vi "WLC fitting_twoside_slope_YCC.vi"(4 "QPD-y":dbl[](array[numeric]), 5 "QPD-x":dbl[](array[numeric]), 6 "Xstage":dbl[](array[numeric]), 7 "T=Read data mode?\nF=Real time fit":bool=TRUE) -> ()   [LabVIEW 2014]
doc: "This VI utilizes the LabVIEW implemented non-linear curve fitting algorithm to fit worm-like chain model. \nThere are 2 modes can be selected: one is real-time fitting mode, the other is data reading mode. \n\nIn the real-time fitting mode, the force-extension assay VI will automatically pass the data and the settings into this VI, and then fitting. \n\nIn the data reading mode, you should first select the data path to read, and manually input all the setting, such as height and fitting range, and then push the \"run\" button. \n\nThe VI will calculate the DNA extension, and extract the pre-set fitting range to do WLC fitting. The data output includes contour length, persistence length, fitted center, recorded data and fitted data."
uses:
  <vilib>/gmath/NI_Gmath.lvlib
  <vilib>/Utility/file.llb/Read From Spreadsheet File (DBL).vi
  <vilib>/Utility/file.llb/Write To Spreadsheet File (DBL).vi
  <vilib>/gmath/NumericalOptimization/Nonlinear Curve Fit LM formula string.vi
panel:
  out "QPD height":dbl
  in  "initial parameters for fit K":dbl[](array[numeric])=[40.0, 1150.0]
  in  "initial parameters 2":dbl[](array[numeric])=[40.0, 1150.0]
  in  "Enum":T1(ring)
  out "residue":dbl
  in  "Tab Control 2":enum32{"Page 1"}(tab)
  in  "T=positive (RHS)\nF=negative (LHS)":bool
  in  "fit only one side?":bool
  in  "OK to fit?":bool
  in  "trap height(nm)":dbl=300.0
  in  "X=T,Y=F":bool=TRUE
  in  "Tab Control":T2(tab)
  out "XY Graph 2":T3(graph)
  out "XY Graph 4":T3(graph)
  out "XY Graph":cluster{"Y":dbl[], "Y":dbl[]}[](graph)
  out "XY Graph 3":cluster{"xDNA-cut":dbl[], "Force-cut":dbl[]}[](graph)
  in  "laser power (mW)":dbl=10.0
  in  "xDNA cut outside (nm)":dbl=2000.0
  in  "stop to save?":bool
  out "yr":dbl
  out "conversion factor (V/um)":dbl=2.6
  in  "center position shift (nm)":dbl=0.0001 format="%_6g"
  in  "center QPD shift mV)":dbl=0.0001 format="%_6g"
  in  "initial parameters for marko":dbl[](array[numeric])=[40.0, 1800.0, 0.001, 0.001]
  out "yi":dbl
  out "Position Array Out":dbl[](array[numeric])
  out "Force constant (pN/nm)":dbl=0.0154
  in  "Length offset":dbl=400.0
  in  "Force offset":dbl=4.0
  in  "F-x data":path
  out "ci":dbl
  out "cr":dbl
  in  "Save fit?":bool
  out "QPD signal Out":dbl[](array[numeric])
  out "position-QPD":T4(graph)
  in  "bead radius(nm)":dbl=515.0
  out "best fit parameters":dbl[](array[numeric])
  # "Lp"
  # "L0"
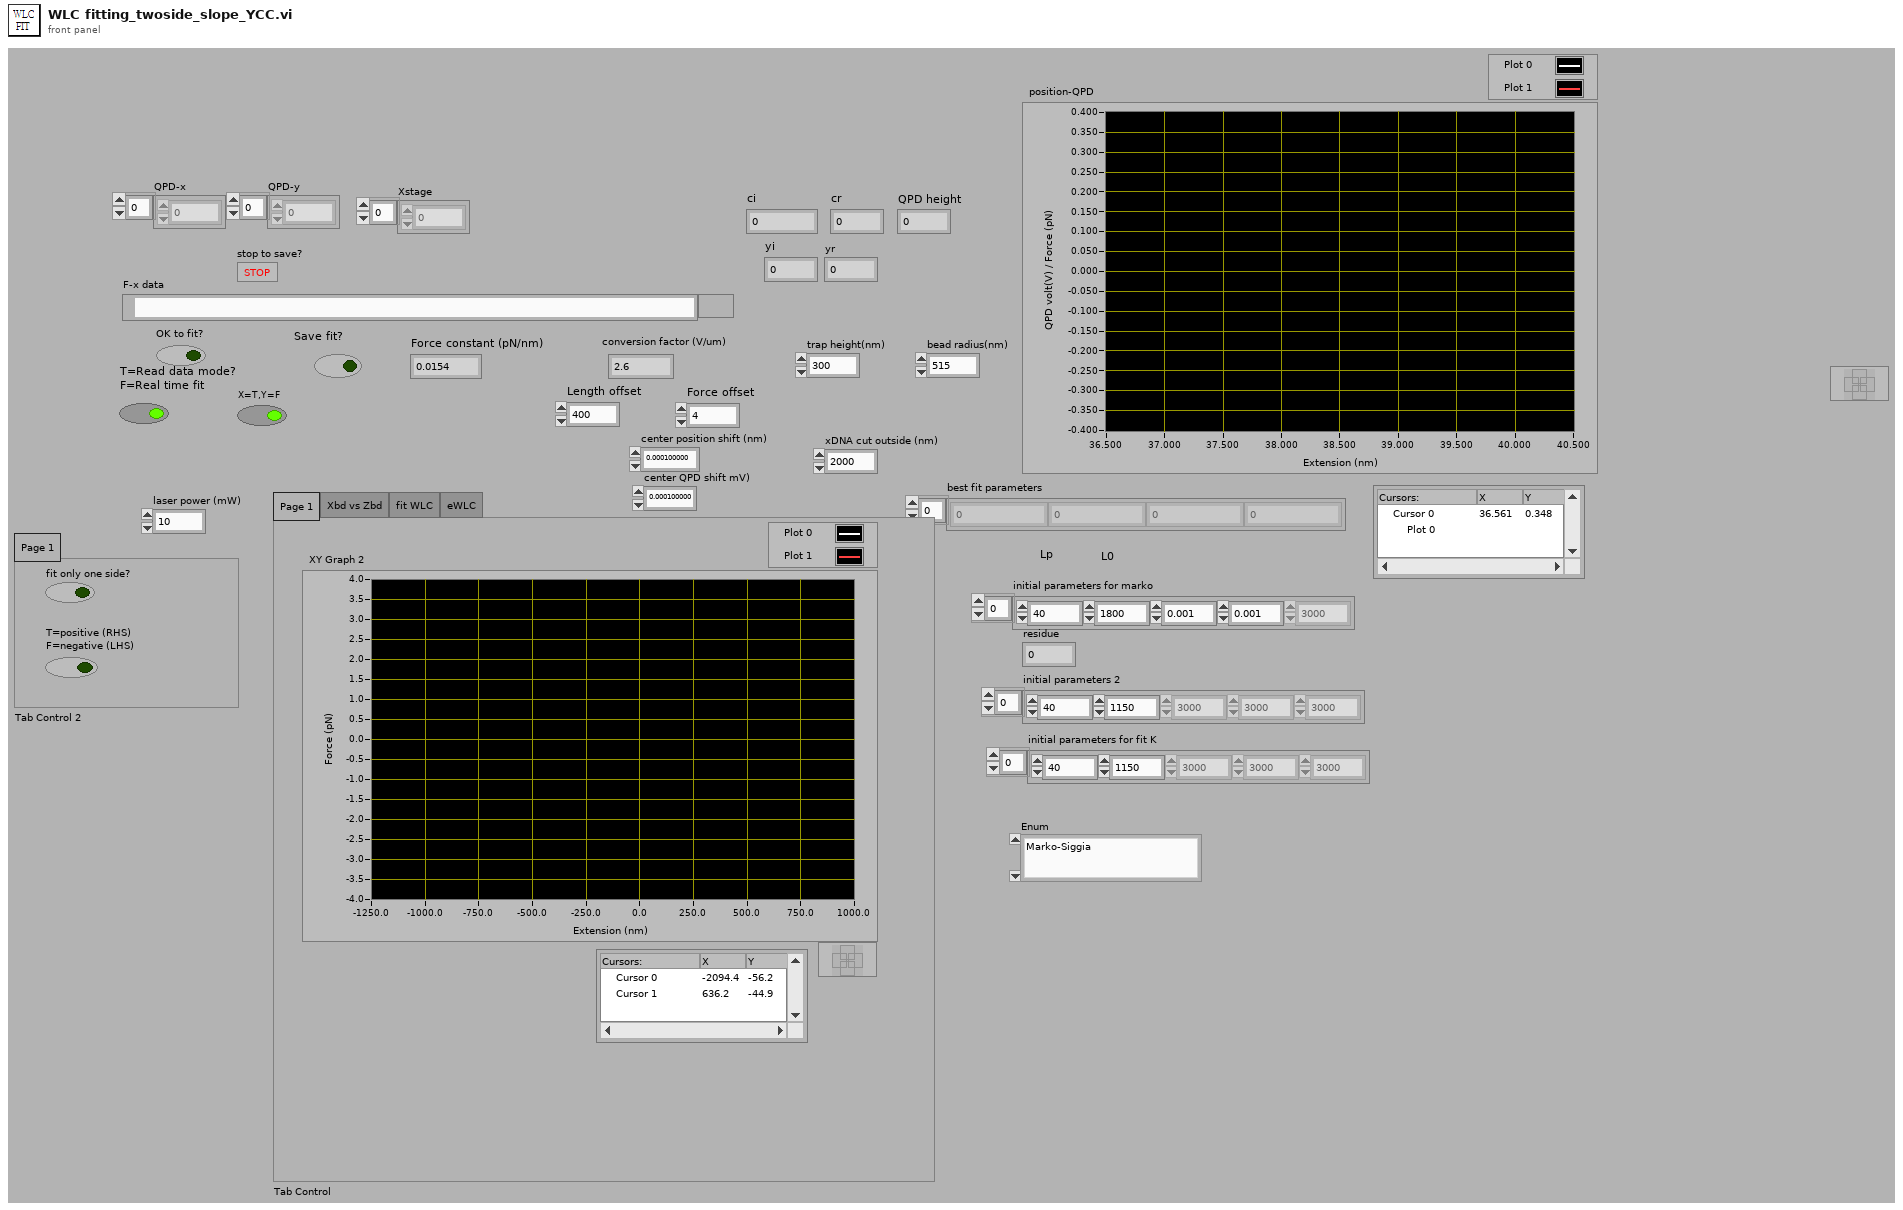
[diagram p1: front panel]
types:
  T1 = enum16{"Marko-Siggia", "modified Marko", "eWLC", "eWLC-modified M-S", "K fit eWLC-modified M-S"}
  T2 = enum32{"Page 1", "Xbd vs Zbd", "fit WLC", "eWLC"}
  T3 = cluster{"cut-full xDNA":dbl[], "cut-full Force":dbl[]}
  T4 = cluster{"QPD signal Out":dbl[], "Position Array Out":dbl[]}
  T5 = cluster{"Position Array Out":dbl[], "QPD signal Out":dbl[]}
  T6 = cluster{"model":string, "Parameters":string[], "x":string}
  T7 = cluster{"xDNA-cut":dbl[], "best nonlinear fit":dbl[]}
  T8 = cluster{"best nonlinear fit":dbl[], "Force-cut":dbl[]}
  T9 = cluster{"xDNA-cut":dbl[], "best nonlinear fit":dbl[]}[]
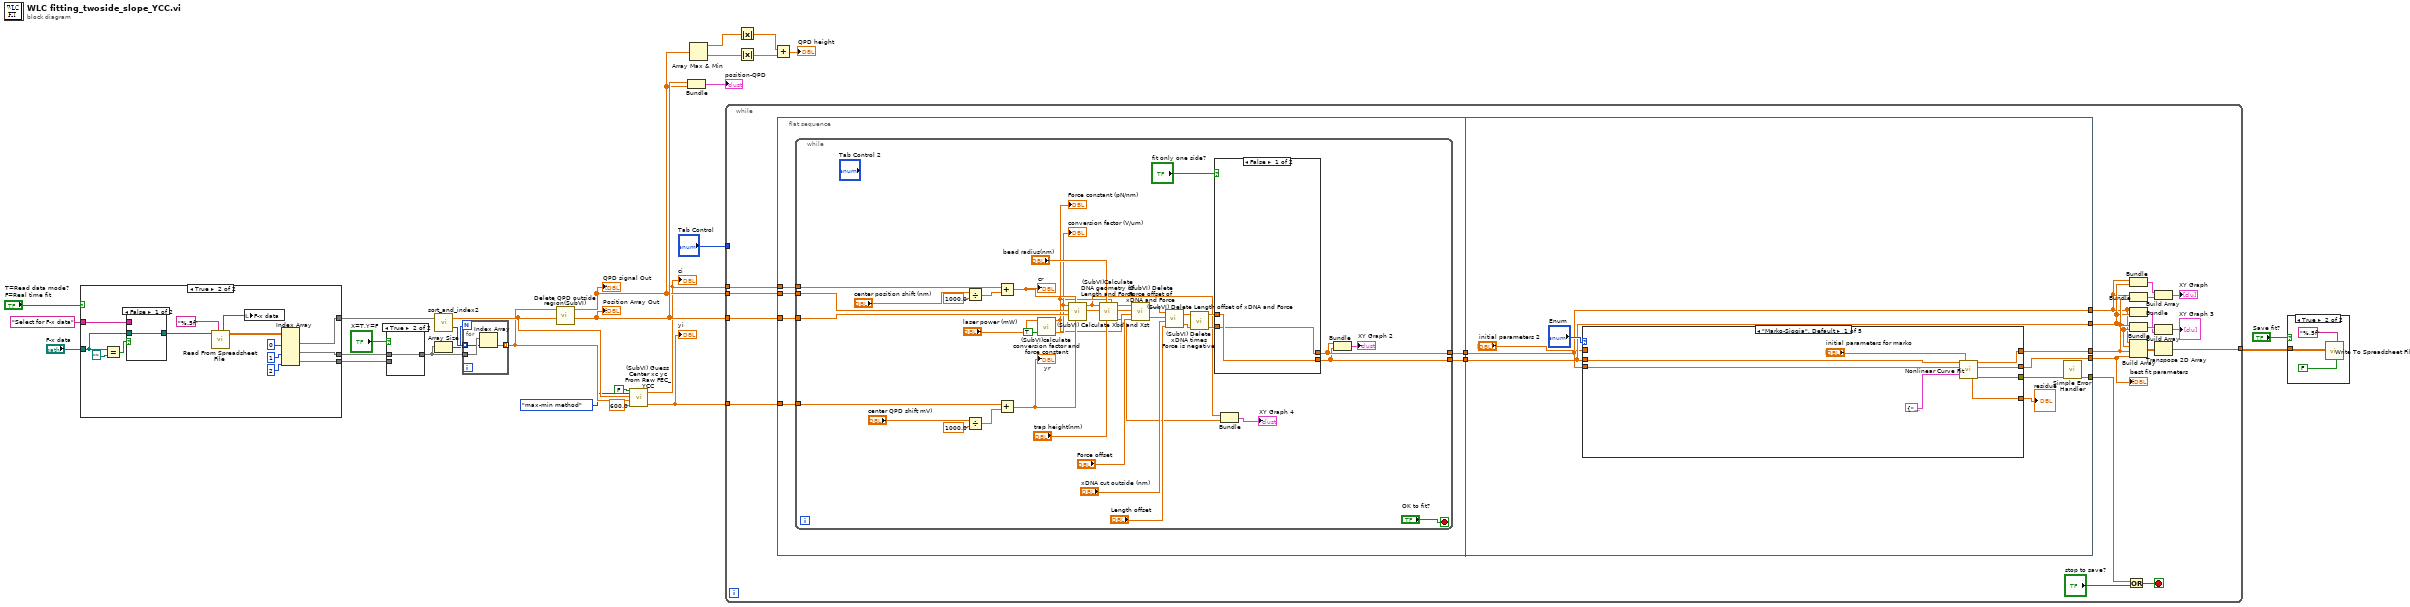
[diagram p0: block diagram]
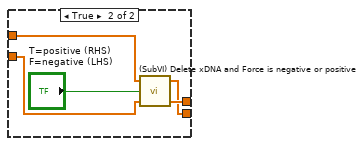
[diagram p2: hidden frame]
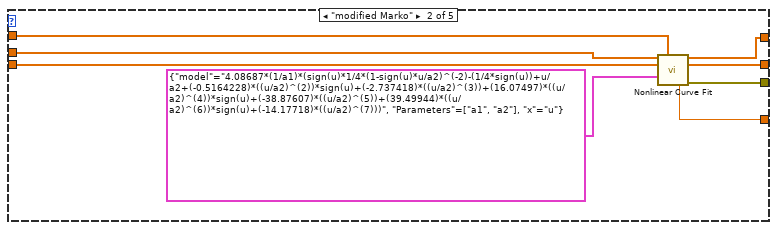
[diagram p3: hidden frame]
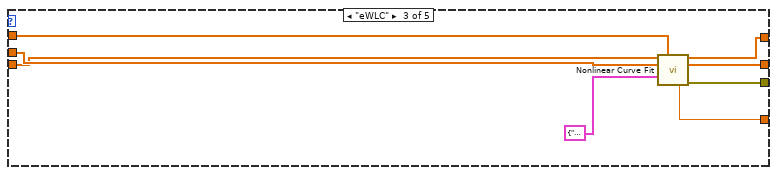
[diagram p4: hidden frame]
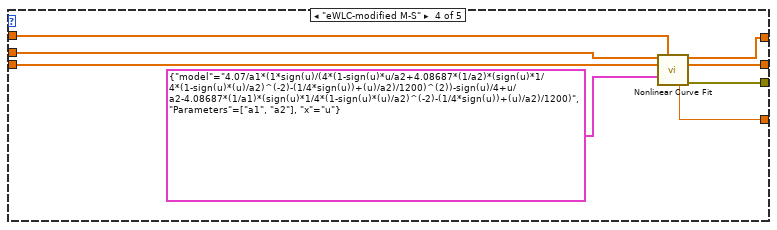
[diagram p5: hidden frame]
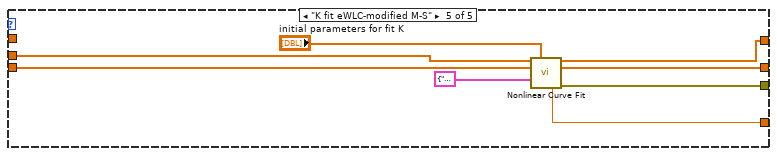
[diagram p6: hidden frame]
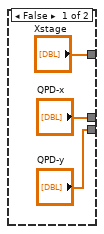
[diagram p8: hidden frame]
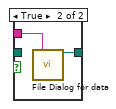
[diagram p9: hidden frame]
diagram:
  n1 = case shown="True" "T=Read data mode?\nF=Real time fit" {
    tunnel: ["QPD-x" w39] -> w27
    tunnel: ["QPD-y" w40] -> w26
    tunnel: ["Xstage" w41] -> w20
    tunnel: "Select for F-x data" ("default name") -> [_ w36]
    tunnel: "F-x data" -> [_ w33]
    frame False {
    }
    frame True {
      n2 = Equal?(x=w33, y=path "") -> (x = y?=w34:bool)
      n3 = case shown="False" w34 {
        tunnel: [w46 w47] -> w37
        tunnel: w36 -> [_ w48]
        tunnel: w33 -> [w46 _]
        frame False {
        }
        frame True {
          n4 = call "File Dialog for data"("prompt"=w48) -> ("selected path"=w47:path)  [unwired: 11 in, 3 out]
        }
      }
      n5 = call-poly <vilib>:"Read From Spreadsheet File.vi"("format (%.3f)"="%.5f", "file path (dialog if empty)"=w37) -> ("all rows"=w45:dbl[][], "new file path (Not A Path if cancelled)"=w32:path)  [unwired: 5 in, 3 out]
      n6 = local write "F-x data"(w32) -> ()
      n7 = Index Array(array=w45, index (col) #1=0 ("disabled index (col)"), index (col) #2=1 ("index (col)"), index (col) #3=2 ("index (col)")) -> (element #1=w41:dbl[], element #2=w39:dbl[], element #3=w40:dbl[])  [unwired: 3 in]
    }
  }
  n8 = case shown="True" "X=T,Y=F" {
    tunnel: w26 -> [w49 _]
    tunnel: [w49 w50] -> w18
    tunnel: w27 -> [_ w50]
    frame False {
    }
    frame True {
    }
  }
  n9 = call "sort_and_index2.vi"("Presorted Array"=w20) -> ("Index"=w19:i32[], "Sorted Array"=w6:dbl[])  [unwired: 1 in]
  n10 = Array Size(array=w18) -> (size(s)=w17:i32)
  n11 = for {
    N: w17 -> [_]
    tunnel: w18 -> [w53]
    tunnel: w19 -> [w52] mode=indexing
    tunnel: [w51] -> w5 mode=indexing
    n12 = Index Array(array=w53, index=w52) -> (element=w51:dbl)
  }
  n13 = call "Delete QPD outside region(SubVI).vi"("Position Array In"=w6, "QPD signal In"=w5) -> ("Position Array Out"=w16:dbl[], "QPD signal Out"=w15:dbl[])  [unwired: 8 in]
  "QPD signal Out" <- w15
  "Position Array Out" <- w16
  n14 = call "(SubVI) Guess Center xc yc From Raw FEC_YCC.vi"("Read data?"=FALSE, "Enum"=enum16{"parity method", "max-min method"}."max-min method", "Stage array(um)"=w6, "QPD array (V)"=w5, "avg range for QPD center (nm)"=600.0) -> ("Guess-stage-center (um)"=w3:dbl, "Guess-QPD-center (V)"=w2:dbl)  [unwired: 2 in]
  "ci" <- w3
  "yi" <- w2
  n15 = Bundle("Position Array Out"=w16, "QPD signal Out"=w15) -> (→"position-QPD":T5)  [unwired: 1 in]
  n16 = Array Max & Min(array=w15) -> (max value=w12:dbl, min value=w11:dbl)  [unwired: 2 out]
  n17 = while {
    tunnel: [w73] -> w23
    tunnel: w16 -> [w71]
    tunnel: w15 -> [w69]
    tunnel: w3 -> [w68]
    tunnel: w2 -> [w67]
    tunnel: "Tab Control" -> [_]
    stop <- w65 stop-if-true
    n18 = flat-sequence {
      tunnel: w71 -> [w80]
      tunnel: w69 -> [w79]
      tunnel: w68 -> [w78]
      tunnel: w67 -> [w77]
      tunnel: [w76] -> w64
      tunnel: [w75] -> w63
      tunnel: [w133] -> w56
      tunnel: w64 -> [w131]
      tunnel: w63 -> [w133]
      tunnel: [w132] -> w59
      tunnel: [w131] -> w57
      tunnel: [w130] -> w62
      tunnel: [w128] -> w61
      frame #0 {
        n19 = while {
          tunnel: w80 -> [w118]
          tunnel: w79 -> [w115]
          tunnel: w78 -> [w114]
          tunnel: w77 -> [w113]
          tunnel: [w95] -> w76
          tunnel: [w96] -> w75
          stop <- "OK to fit?" stop-if-true
          n20 = Divide(x="center position shift (nm)", y=1000.0) -> (x/y=w89:dbl)
          n21 = Divide(x="center QPD shift mV)", y=1000.0) -> (x/y=w85:dbl)
          n22 = Add(x=w114, y=w89) -> (x+y=w111:dbl)
          "cr" <- w111
          n23 = Add(x=w113, y=w85) -> (x+y=w112:dbl)
          "yr" <- w112
          n24 = call "(SubVI)calculate conversion factor and force constant.vi"("X=T\nY=F"=TRUE ("X=T\nY=F"), "laser power (mW)"="laser power (mW)") -> ("conversion factor (V/um)"=w106:dbl, "force constant (pN/nm)"=w91:dbl)  [unwired: 2 in]
          "Force constant (pN/nm)" <- w91
          "conversion factor (V/um)" <- w106
          n25 = call "(SubVI) Calculate Xbd and Xst.vi"("yr"=w112, "cr"=w111, "Stage Position"=w118, "QPD signal"=w115, "conversion factor (V/um)"=w106) -> ("Xst"=w93:dbl[], "Xbd"=w81:dbl[])  [unwired: 5 in]
          n26 = call "(SubVI)Calculate DNA geometry of Length and Force.vi"("Force constant (pN/nm)"=w91, "trap height(nm)"="trap height(nm)", "bead radius(nm)"="bead radius(nm)", "Xst"=w93, "Xbd"=w81) -> ("zbd (nm)"=w82:dbl[], "xDNA"=w105:dbl[], "Force"=w104:dbl[])  [unwired: 4 in]
          n27 = call "(SubVI) Delete Force offset of xDNA and Force.vi"("Force offset"="Force offset", "force constant"=w91, "xDNA"=w105, "Force"=w104) -> ("cut-full xDNA"=w101:dbl[], "cut-full Force"=w102:dbl[])
          n28 = call "(SubVI) Delete Length offset of xDNA and Force.vi"("Length offset"="Length offset", "xDNA cut outside (nm)"="xDNA cut outside (nm)", "xDNA"=w101, "Force"=w102) -> ("cut-full xDNA"=w99:dbl[], "cut-full Force"=w100:dbl[])
          n29 = call "(SubVI) Delete xDNA times Force is negative.vi"("xDNA"=w99, "Force"=w100) -> ("xDNA-cut"=w97:dbl[], "Force-cut"=w98:dbl[])  [unwired: 2 in]
          n30 = case shown="False" "fit only one side?" {
            tunnel: w98 -> [w120 w125]
            tunnel: w97 -> [w119 w123]
            tunnel: [w119 w122] -> w96
            tunnel: [w120 w121] -> w95
            frame False {
            }
            frame True {
              n31 = call "(SubVI) Delete xDNA and Force is negative or positive.vi"("xDNA"=w123, "T=positive (RHS)\nF=negative (LHS)"="T=positive (RHS)\nF=negative (LHS)", "Force"=w125) -> ("xDNA-cut"=w122:dbl[], "Force-cut"=w121:dbl[])  [unwired: 1 in]
            }
          }
          n32 = Bundle("Xbd"=w81, "zbd (nm)"=w82) -> (→"XY Graph 4":cluster{"Xbd":dbl[], "zbd (nm)":dbl[]})  [unwired: 1 out]
          n33 = Bundle("xDNA-cut"=w96, "Force-cut"=w95) -> (→"XY Graph 2":cluster{"xDNA-cut":dbl[], "Force-cut":dbl[]})  [unwired: 1 out]
        }
      }
      frame #1 {
        n34 = case shown="\"Marko-Siggia\", Default" "Enum" {
          tunnel: "initial parameters 2" -> [_ w149 w155 w165 _]
          tunnel: w131 -> [w141 w147 w157 w163 w173]
          tunnel: w133 -> [w140 w148 w156 w164 w172]
          tunnel: [w139 w144 w153 w159 w167] -> w132
          tunnel: [w138 w145 w154 w160 w168] -> w130
          tunnel: [w137 w146 w152 w161 w169] -> w129
          tunnel: [w136 w143 w151 w162 w170] -> w127
          frame "Marko-Siggia", Default {
            n35 = call-poly <vilib>:"Nonlinear Curve Fit.vi"("Y"=w141, "initial parameters"="initial parameters for marko", "X"=w140, "model description"=T6 {"model"="4.08687*(1/a1)*(sign(u-a3)*1/4*(1-sign(u-a3)*(u-a3)/a2)^(-2)-(1/4*sign(u-a3))+(u-a3)/a2)+a4", "Parameters"=["a1", "a2", "a3", "a4"], "x"="u"}) -> ("best nonlinear fit"=w139:dbl[], "best fit parameters"=w138:dbl[], "residue"=w136:dbl, "error out"=w137:errorcluster)  [unwired: 3 in, 5 out]
          }
          frame "modified Marko" {
            n36 = call-poly <vilib>:"Nonlinear Curve Fit.vi"("Y"=w147, "initial parameters"=w149, "X"=w148, "model description"=T6 {"model"="4.08687*(1/a1)*(sign(u)*1/4*(1-sign(u)*u/a2)^(-2)-(1/4*sign(u))+u/a2+(-0.5164228)*((u/a2)^(2))*sign(u)+(-2.737418)*((u/a2)^(3))+(16.07497)*((u/a2)^(4))*sign(u)+(-38.87607)*((u/a2)^(5))+(39.49944)*((u/a2)^(6))*sign(u)+(-14.17718)*((u/a2)^(7)))", "Parameters"=["a1", "a2"], "x"="u"}) -> ("best nonlinear fit"=w144:dbl[], "best fit parameters"=w145:dbl[], "residue"=w143:dbl, "error out"=w146:errorcluster)  [unwired: 3 in, 5 out]
          }
          frame "eWLC" {
            n37 = call-poly <vilib>:"Nonlinear Curve Fit.vi"("Y"=w156, "initial parameters"=w155, "X"=w157, "model description"=T6 {"model"="a2*(1*sign(u)-sign(u)*1/2*(4.07/u/a1)^(0.5)+sign(u)*u/1200)", "Parameters"=["a1", "a2"], "x"="u"}) -> ("best nonlinear fit"=w153:dbl[], "best fit parameters"=w154:dbl[], "residue"=w151:dbl, "error out"=w152:errorcluster)  [unwired: 3 in, 5 out]
          }
          frame "eWLC-modified M-S" {
            n38 = call-poly <vilib>:"Nonlinear Curve Fit.vi"("Y"=w163, "initial parameters"=w165, "X"=w164, "model description"=T6 {"model"="4.07/a1*(1*sign(u)/(4*(1-sign(u)*u/a2+4.08687*(1/a2)*(sign(u)*1/4*(1-sign(u)*(u)/a2)^(-2)-(1/4*sign(u))+(u)/a2)/1200)^(2))-sign(u)/4+u/a2-4.08687*(1/a1)*(sign(u)*1/4*(1-sign(u)*(u)/a2)^(-2)-(1/4*sign(u))+(u)/a2)/1200)", "Parameters"=["a1", "a2"], "x"="u"}) -> ("best nonlinear fit"=w159:dbl[], "best fit parameters"=w160:dbl[], "residue"=w162:dbl, "error out"=w161:errorcluster)  [unwired: 7 in, 1 out]
          }
          frame "K fit eWLC-modified M-S" {
            n39 = call-poly <vilib>:"Nonlinear Curve Fit.vi"("Y"=w173, "initial parameters"="initial parameters for fit K", "X"=w172, "model description"=T6 {"model"="4.07/a1*(1*sign(u)/(4*(1-sign(u)*u/a2+4.08687*(1/a2)*(sign(u)*1/4*(1-sign(u)*(u)/a2)^(-2)-(1/4*sign(u))+(u)/a2)/a3)^(2))-sign(u)/4+u/a2-4.08687*(1/a1)*(sign(u)*1/4*(1-sign(u)*(u)/a2)^(-2)-(1/4*sign(u))+(u)/a2)/a3)", "Parameters"=["a1", "a2", "a3"], "x"="u"}) -> ("best nonlinear fit"=w167:dbl[], "best fit parameters"=w168:dbl[], "residue"=w170:dbl, "error out"=w169:errorcluster)  [unwired: 7 in, 1 out]
          }
        }
        "residue" <- w127
        n40 = call <vilib>:"Simple Error Handler.vi"("error in (no error)"=w129) -> ("error out"=w128:errorcluster)  [unwired: 4 in, 4 out]
      }
    }
    n41 = Or(x=w61, y="stop to save?") -> (x .or. y?=w65:bool)
    n42 = Bundle("xDNA-cut"=w56, "Force-cut"=w57) -> (w72:cluster{"xDNA-cut":dbl[], "Force-cut":dbl[]})  [unwired: 1 out]
    n43 = Bundle("xDNA-cut"=w56, "best nonlinear fit"=w59) -> (w70:T7)  [unwired: 1 out]
    n44 = Bundle("xDNA-cut"=w56, "Force-cut"=w57) -> (w55:cluster{"xDNA-cut":dbl[], "Force-cut":dbl[]})  [unwired: 1 out]
    n45 = Bundle("best nonlinear fit"=w59, "Force-cut"=w57) -> (w58:T8)  [unwired: 1 out]
    n46 = Build Array(w56, w57, w59, w62) -> (w74:dbl[][])
    n47 = Build Array(w72, w70) -> (→"XY Graph":T9)
    n48 = Build Array(w58, w55) -> (→"XY Graph 3":cluster{"xDNA-cut":dbl[], "Force-cut":dbl[]}[])
    n49 = Transpose 2D Array(2D array=w74) -> (transposed array=w73:dbl[][])
    "best fit parameters" <- w62
  }
  n50 = Absolute Value(x=w12) -> (abs(x)=w10:dbl)
  n51 = Absolute Value(x=w11) -> (abs(x)=w9:dbl)
  n52 = Add(x=w10, y=w9) -> (x+y=→"QPD height":dbl)
  n53 = case shown="True" "Save fit?" {
    tunnel: w23 -> [_ w175]
    frame False {
    }
    frame True {
      n54 = call-poly <vilib>:"Write To Spreadsheet File.vi"("transpose? (no:F)"=FALSE, "format (%.3f)"="%.5f", "2D data"=w175) -> ()  [unwired: 5 in, 1 out]
    }
  }
